vi "ReadXmlFileProperties.vi"(3 "error in":errorcluster, 4 "NameFileAndType":string, 5 "parameters":variant) -> (0 "error out":errorcluster, 1 "OutputParamReadFile":variant, 2 "PathXMLFile":path)   [LabVIEW 2016]
uses:
  <vilib>/Utility/xml.llb/Read From XML File(string).vi
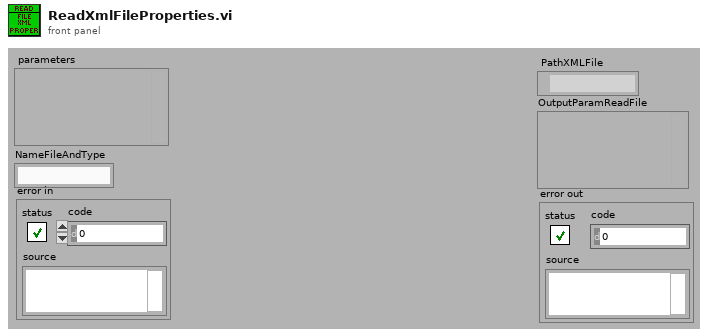
[diagram p1: front panel]
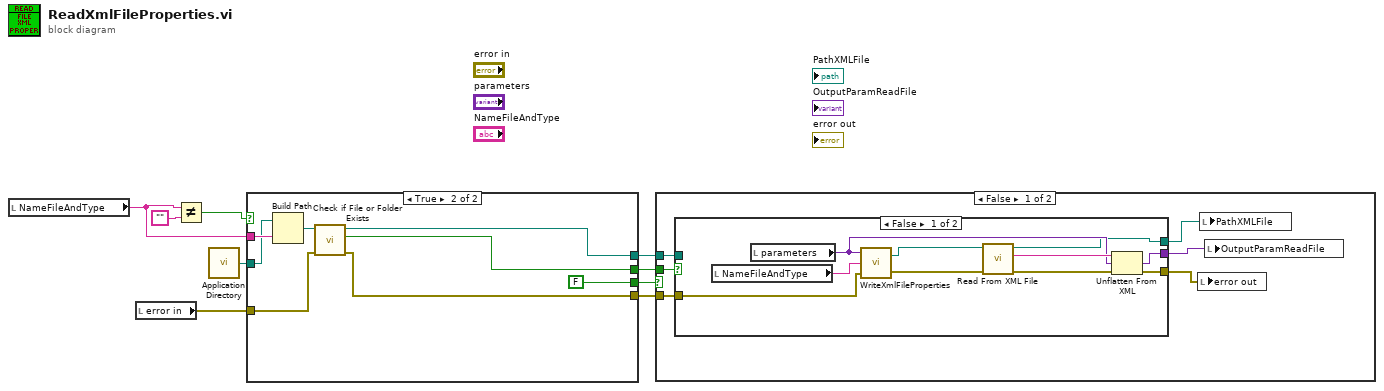
[diagram p0: block diagram]
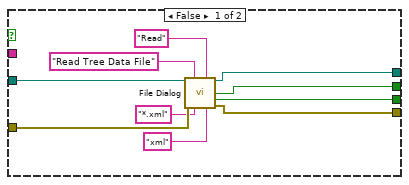
[diagram p2: hidden frame]
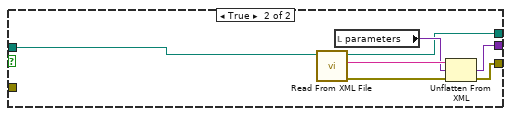
[diagram p3: hidden frame]
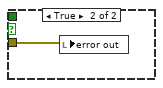
[diagram p4: hidden frame]
diagram:
  n1 = local read "NameFileAndType"() -> (w2:string)
  n2 = local read "error in"() -> (w6:errorcluster)
  n3 = Not Equal?(x=w2, y="") -> (x != y?=w3:bool)
  n4 = call <vilib>:"Application Directory.vi"() -> ("Application Directory"=w5:path)
  n5 = case shown="True" w3 {
    tunnel: [w17 w27] -> w9
    tunnel: [w14 w26] -> w8
    tunnel: w2 -> [_ w24]
    tunnel: [w16 w23] -> w7
    tunnel: w6 -> [w18 w22]
    tunnel: w5 -> [w19 w21]
    tunnel: [w15 FALSE ("cancelled")] -> w4
    frame False {
      n6 = call "File Dialog"("start path"=w19, "prompt"="Read Tree Data File", "button label"="Read", "error in"=w18, "pattern (all files)"="*.xml", "pattern label"="xml") -> ("selected path"=w17:path, "exists"=w14:bool, "cancelled"=w15:bool, "error out"=w16:errorcluster)  [unwired: 6 in]
    }
    frame True {
      n7 = Build Path(base path=w21, name or relative path=w24) -> (appended path=w25:path)
      n8 = call <vilib>:"Check if File or Folder Exists.vi"("error in (no error)"=w22, "path"=w25) -> ("error out"=w23:errorcluster, "file or folder exists?"=w26:bool, "dup path"=w27:path)  [unwired: 7 in]
    }
  }
  n9 = case shown="False" w4 {
    tunnel: w9 -> [w33 _]
    tunnel: w8 -> [w32 _]
    tunnel: w7 -> [w28 w51]
    frame False {
      n10 = case shown="False" w32 {
        tunnel: w33 -> [_ w49]
        tunnel: [w37 w46] -> w31
        tunnel: [w36 w45] -> w30
        tunnel: [w35 w44] -> w29
        tunnel: w28 -> [w34 _]
        frame False {
          n11 = local read "NameFileAndType"() -> (w39:string)
          n12 = local read "parameters"() -> (w38:variant)
          n13 = call "WriteXmlFileProperties.vi"("error in"=w34, "NameFileAndType"=w39, "Parameters"=w38) -> ("error out"=w40:errorcluster, "PathXMLFile"=w41:path)
          n14 = call-poly <vilib>:"Read From XML File.vi"("error in (no error)"=w40, "XML File Path"=w41) -> ("error out"=w42:errorcluster, "XML Elements"=w43:string, "XML File Path(duplicate)"=w36:path)  [unwired: 7 in]
          n15 = Unflatten From XML(xml string=w43, type=w38, error in (no error)=w42) -> (value=w37:variant, error out=w35:errorcluster)
        }
        frame True {
          n16 = call-poly <vilib>:"Read From XML File.vi"("XML File Path"=w49) -> ("error out"=w50:errorcluster, "XML Elements"=w48:string, "XML File Path(duplicate)"=w45:path)  [unwired: 8 in]
          n17 = local read "parameters"() -> (w47:variant)
          n18 = Unflatten From XML(xml string=w48, type=w47, error in (no error)=w50) -> (value=w46:variant, error out=w44:errorcluster)
        }
      }
      n19 = local write "error out"(w29) -> ()
      n20 = local write "PathXMLFile"(w30) -> ()
      n21 = local write "OutputParamReadFile"(w31) -> ()
    }
    frame True {
      n22 = local write "error out"(w51) -> ()
    }
  }
